vi "UMLEditor_PackageClasses.vi"(0 "DiagramIn":refnum<class "Graph.lvclass">, 3 "Settings":T1={"Levels"=-1}, 5 "error in (no error)":errorcluster) -> (19 "error out":errorcluster)   [LabVIEW 2020]
doc: "Gets current diagram values"
uses:
  <resource>/Framework/Providers/Open_GDS/UML/UMLEditor/UMLEditor_PackageClasses.ctl
  <resource>/Framework/Providers/Open_GDS/UML/Graph_class/Graph.lvclass
  <resource>/Framework/Providers/Open_GDS/UML/Graphics_class/FontType.ctl
  <resource>/Framework/Providers/Open_GDS/UML/UMLEditor/UMLEditor BusyDialogAction.ctl
  <resource>/Framework/Providers/Open_GDS/UML/ClassNode_class/ClassNode.lvclass
  C:/Program Files (x86)/National Instruments/LabVIEW 2020/resource/Framework/Providers/Open_GDS/UML/AbstractNode_class/AbstractNode.lvclass
  <resource>/Framework/Providers/Open_GDS/UML/PackageNode_class/PackageNode.lvclass
  C:/Program Files (x86)/National Instruments/LabVIEW 2020/resource/Framework/Providers/Open_GDS/UML/RectangularNode_class/RectangularNode.lvclass
  <resource>/Framework/Providers/Open_GDS/UML/ContextHelp/ContextHelp_HelpTexts.ctl
  <resource>/Framework/Providers/Open_GDS/UML/General/Point/Point Point2D.ctl
  <resource>/Framework/Providers/Open_GDS/UML/RectangularNode_class/RectangularNode.lvclass
  <resource>/Framework/Providers/Open_GDS/UML/Graphics_class/Graphics.lvclass
  <resource>/Framework/Providers/Open_GDS/UML/AbstractNode_class/AbstractNode.lvclass
panel:
  in  "MoveNodes":bool
  in  "Levels":i32=3 caption="Maximum levels of packages to create" min=1 max=100
  in  "Help":bool
  in  "cancel":bool
  in  "ok":bool
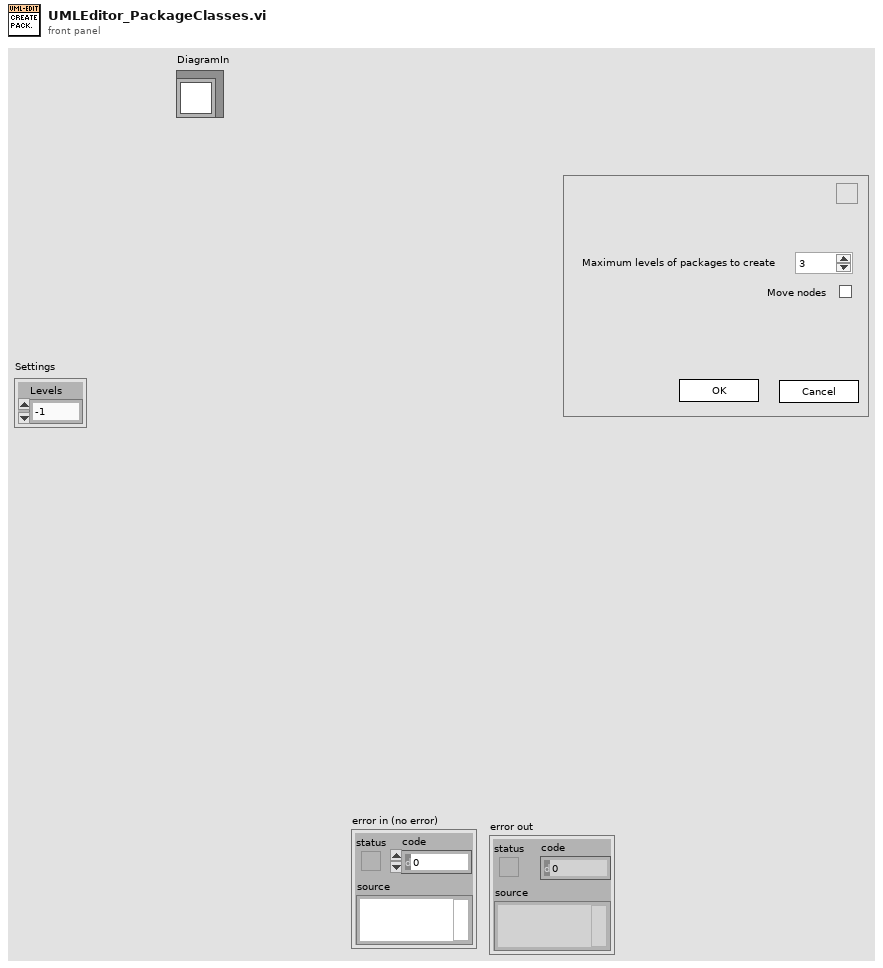
[diagram p1: front panel]
types:
  T1 = typedef "UMLEditor_PackageClasses.ctl" = cluster{"Levels":i32}
  T2 = cluster{"ClassNodes":refnum<class "ClassNode.lvclass">[], "Folders":cluster{"Foldername":string, "Path":path, "Nodes":refnum<class "ClassNode.lvclass">[], "SubFolders":path[], "PackageNode":refnum<class "PackageNode.lvclass">}[], "PackageNames":string[], "PackagesNodes":refnum<class "PackageNode.lvclass">[]}
  T3 = typedef "UMLEditor BusyDialogAction.ctl" = enum16{"Initialize", "Open(VIs)", "Open(i)", "Send_I-Value", "SendStatusMessage", "GetBusyDialogStatus", "Close", "Quit"}
  T4 = typedef "Graphics.lvclass/FontType.ctl" = cluster{"Font Name:":string, "Size":i16, "Strikeout?":bool, "Italic?":bool, "Underline?":bool, "Outline?":bool, "Shadow?":bool, "Bold?":bool}
  T5 = typedef "ContextHelp_HelpTexts.ctl" = enum16{"None(Hide)", "Default", "Help", "Welcome", "GettingStarted", "ClassDiagram_Help", "SequenceDiagram_Help", "UseCaseDiagram_Help", "BSelect", "BClass", "BInterface", "BPackage", "BNote", "BDependency", "BInheritance", "BInterfaceImplementation", "BAssociation", "BAggregation", "BCompAggregation", "BNoteConnector", "BObject", "BActionBar", "BCall", "BSystem", "BActor", "BUseCase", "BGeneralization", "BIncludes", "BExtends", "BUseCaseDiagramAssociation", "ClassRelationshipEdge editDialog_Bent Style", "ClassRelationshipEdge editDialog_RelationType", "ClassRelationshipEdge editDialog_Reverse association", "ClassRelationshipEdge editDialog_Start label", "ClassRelationshipEdge editDialog_Middle label", "ClassRelationshipEdge editDialog_End label", "UMLEditor reversedEngineering_Pathes", "ReversedEngineering StateReverseDialog_Help", "ReversedEngineering StateQueuedSettings_Help", "UMLEditor reversedEngineering_AddTopVIs", "UMLEditor reversedEngineering_AddClasses", "UMLEditor reversedEngineering_AddDirs", "UMLEditor reversedEngineering_Recursively", "UMLEditor reversedEngineering_Remove", "UMLEditor reversedEngineering_ClearList", "UMLEditor reversedEngineering_HideSubAss", "UMLEditor reversedEngineering_CreateTypes", "UMLEditor reversedEngineering_OnlyInheritance", "UMLEditor reversedEngineering_CreateApplication", "UMLEditor reversedEngineering_OK", "UMLEditor reversedEngineering_Cancel", "UMLEditor reversedEngineering_Help", "UMLEditor createWizardScriptFile_ScriptfilePath", "UMLEditor createWizardScriptFile_ClassPath", "UMLEditor createWizardScriptFile_Use", "UMLEditor createWizardScriptFile_PrivateDirName", "UMLEditor createWizardScriptFile_DirAppend", "UMLEditor createWizardScriptFile_Separator Character", "UMLEditor createWizardScriptFile_OK", "UMLEditor createWizardScriptFile_Cancel", "UMLEditor createWizardScriptFile_Help", "ClassNode editDialog_Class Name", "InterfaceNode editDialog_Class Name", "ClassNode editDialog_Attribute", "ClassNode editDialog_Methods", "InterfaceNode editDialog_Methods", "ClassNode editDialog_connection", "InterfaceNode editDialog_connection", "ClassNode editDialog_StereoType", "ClassNode editDialog_ShowAttrib", "ClassNode editDialog_ShowMethods", "ClassNode editDialog_ClassPath", "ClassNode editDialog_AddAttribute", "ClassNode editDialog_AddMethod", "InterfaceNode editDialog_AddMethod", "ClassNode AttributeGuide_AttributeName", "ClassNode AttributeGuide_Array?", "ClassNode AttributeGuide_Data Type", "ClassNode AttributeGuide_RefName", "ClassNode AttributeGuide_Preview", "ClassNode AttributeGuide_OK", "ClassNode AttributeGuide_Cancel", "ClassNode MethodGuide_Visibility", "ClassNode MethodGuide_Method Name", "ClassNode MethodGuide_Preview", "ClassNode MethodGuide_OK", "ClassNode MethodGuide_Cancel", "CallNode EditCallProperties_AllButtons", "ObjectNode EditObjectlProperties_AllButtons", "ActorNode EditActorProperties_AllButtons", "UseCaseRelationshipNode EditUseCaselProperties_AllButtons", "UseCaseNode EditUseCaselProperties_AllButtons", "SystemNode EditSystemProperties_AllButtons", "ReversedEngineering UpdateAttributes_AllButtons", "StateNode editDialog_AllButtons", "StateTransition editDialog_AllButtons", "ArrangeNodes Main_Picture", "ArrangeNodes Main_Zoom", "ArrangeNodes Main_Auto Zoom", "ArrangeNodes Main_shorten", "ArrangeNodes Main_Min Length", "ArrangeNodes Main_Max Length", "ArrangeNodes Main_increase", "ArrangeNodes Main_decrease", "ArrangeNodes Main_Shake", "ArrangeNodes Main", "BState", "BInitialState", "BFinalState", "BStateTransition", "StateDiagram_Help", "StateDiagram_PropertiesAllButtons", "ReversedEngineering StateReverseDialog_ClearStates", "ReversedEngineering StateReverseDialog_UseQueuedStateMachines", "ReversedEngineering StateReverseDialog_QueuedSettings", "ReversedEngineering StateReverseDialog_SearchForVIs", "ReversedEngineering StateReverseDialog_SearchCriteria", "OptionsDialog_ClassBasePath", "OptionsDialog_VIPath", "OptionsDialog_ApplicationPath", "OptionsDialog_WizDir", "OptionsDialog_IniFilePath", "OptionsDialog_DefineColors", "OptionsDialog_Help", "OptionsDialog_CreateTypes", "ClassRelationshipEdge editDialog_SplitWire"}
  T6 = typedef "Point Point2D.ctl" = cluster{"x":dbl, "y":dbl}
  T7 = typedef "ContextHelp_ShowType.ctl" = cluster{"Header":string, "Picture":picture, "Text":string}
  T8 = cluster{"Foldername":string, "Path":path, "Nodes":refnum<class "ClassNode.lvclass">[], "SubFolders":path[], "PackageNode":refnum<class "PackageNode.lvclass">}
  T9 = cluster{"Foldername":string, "Path":path, "Nodes":refnum<class "ClassNode.lvclass">[], "SubFolders":path[], "PackageNode":refnum<class "PackageNode.lvclass">}[]
  T10 = typedef "Rectangle Rectangle2D.ctl" = cluster{"x":dbl, "y":dbl, "width":dbl, "height":dbl}
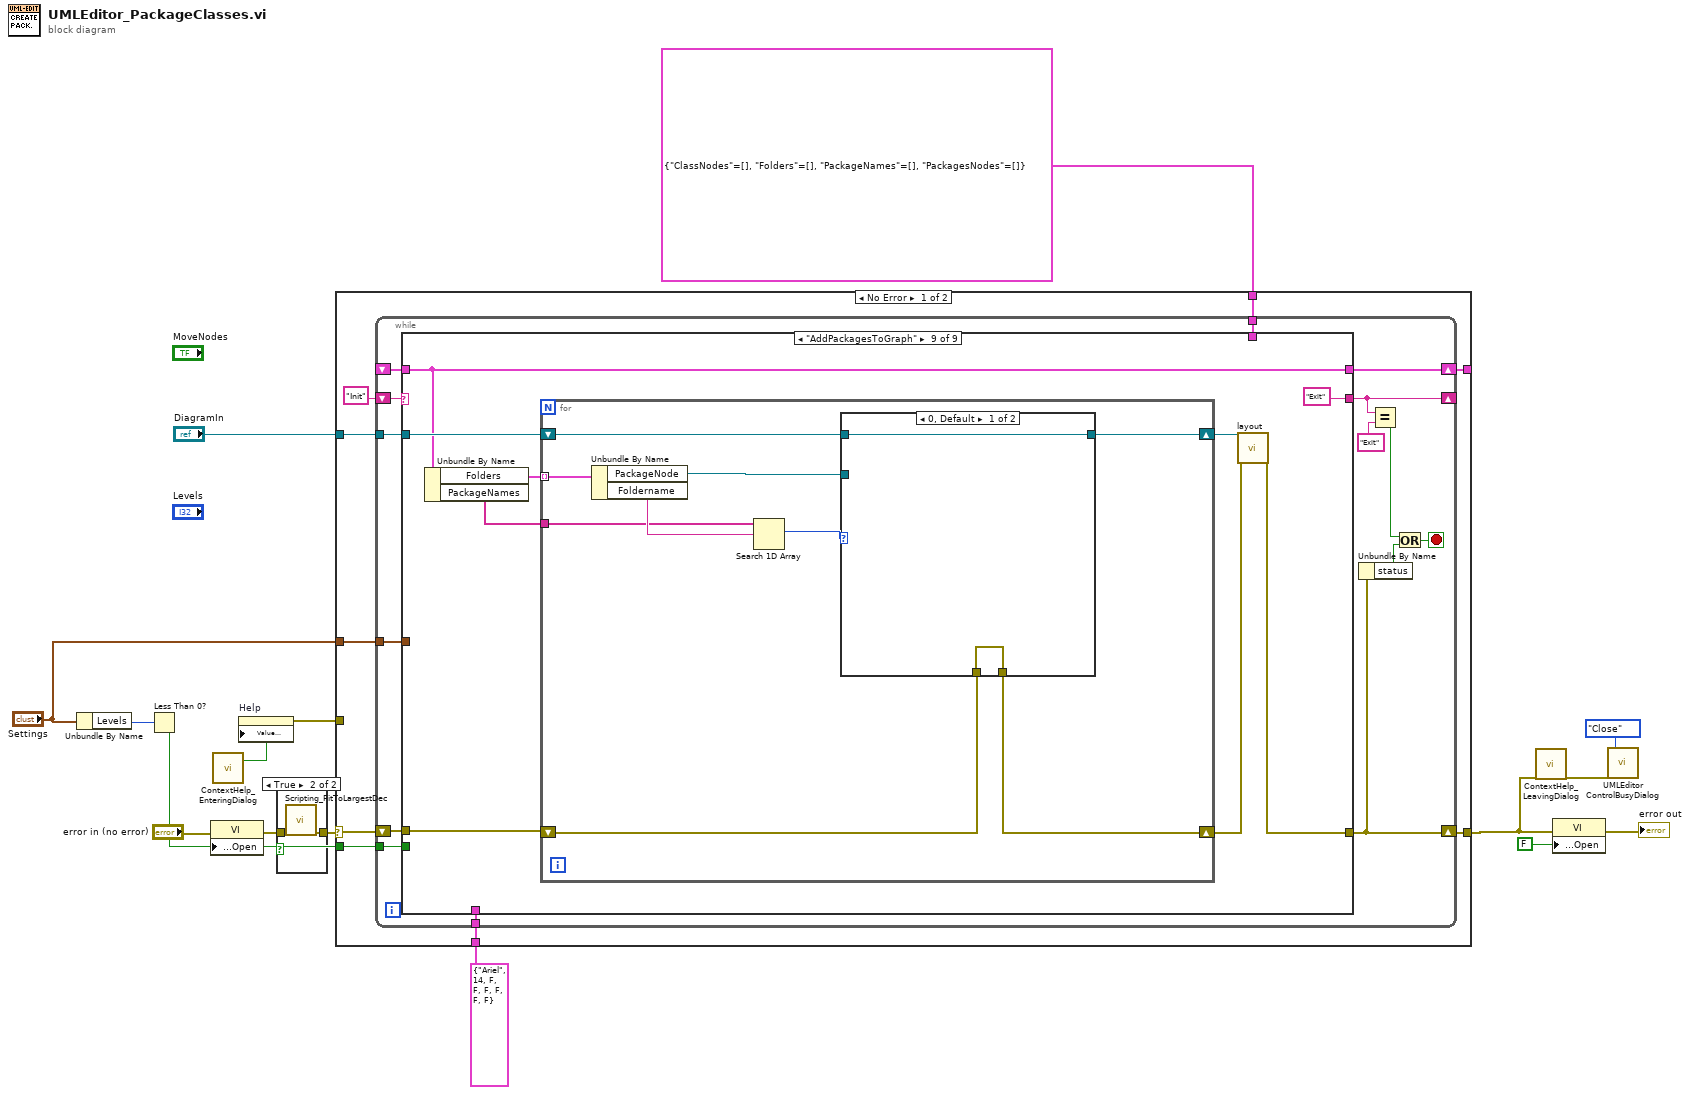
[diagram p0: block diagram]
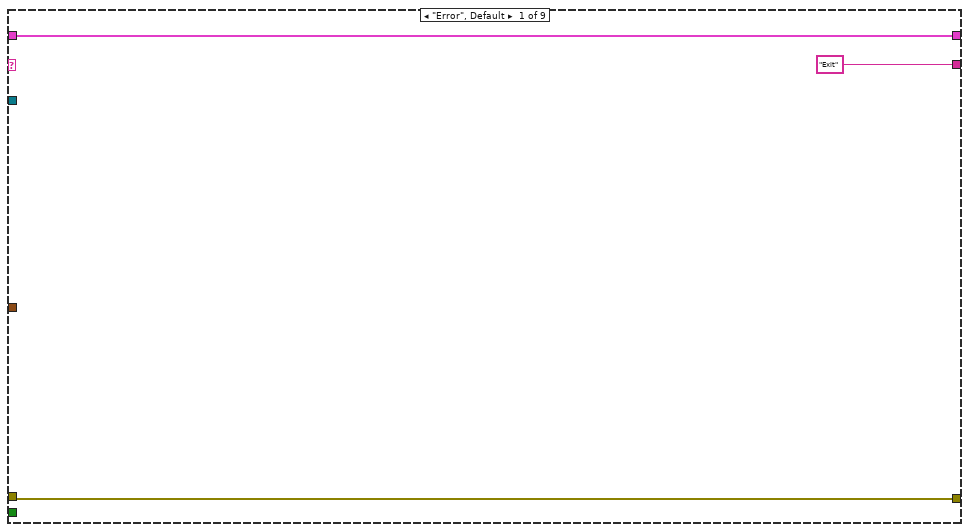
[diagram p3: hidden frame]
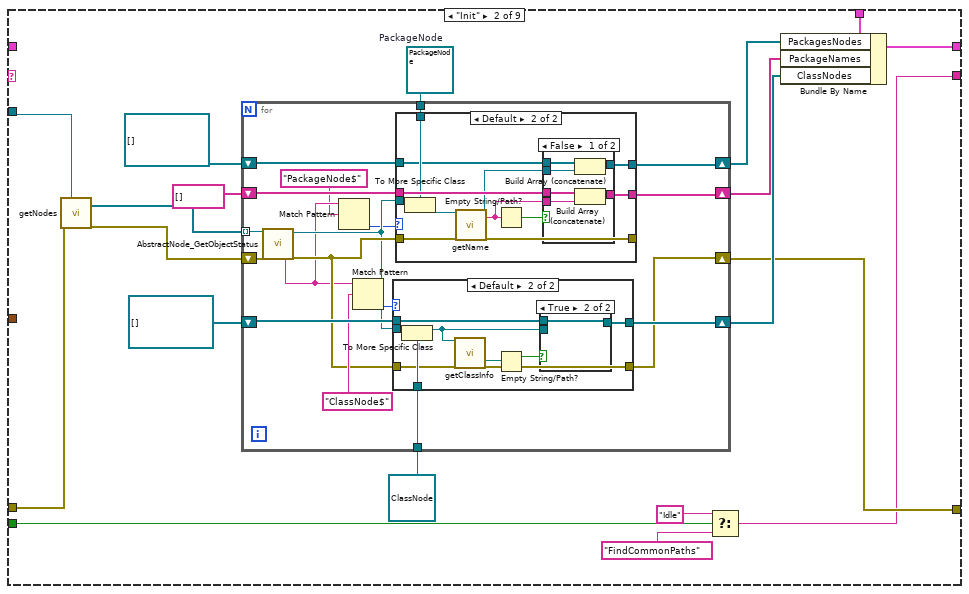
[diagram p4: hidden frame]
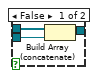
[diagram p8: hidden frame]
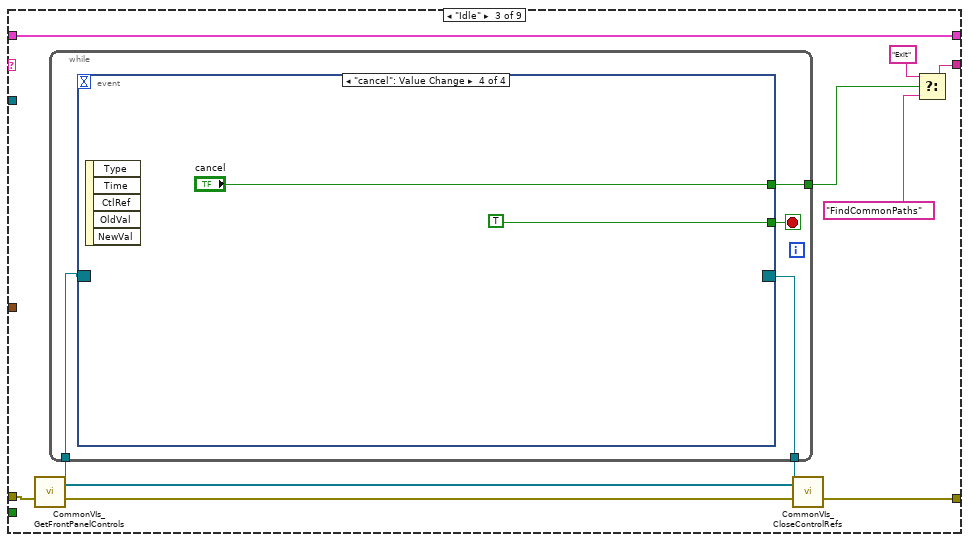
[diagram p9: hidden frame]
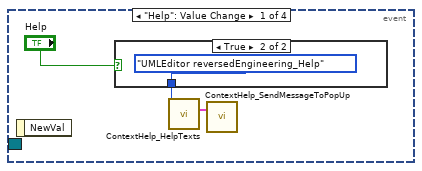
[diagram p10: hidden frame]
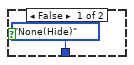
[diagram p11: hidden frame]
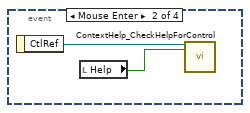
[diagram p12: hidden frame]
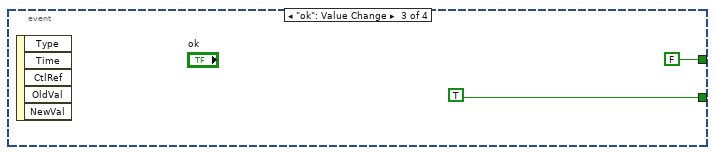
[diagram p13: hidden frame]
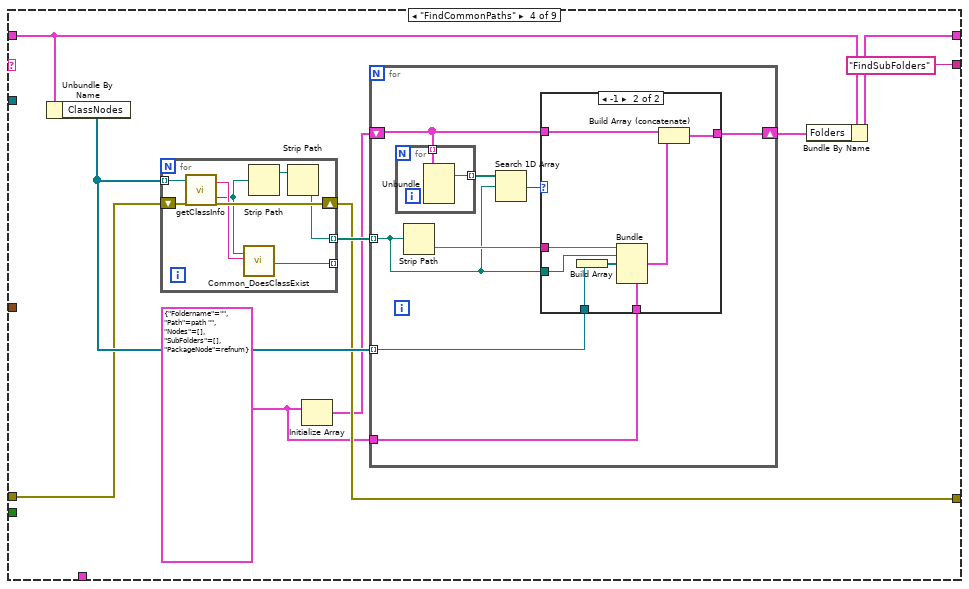
[diagram p14: hidden frame]
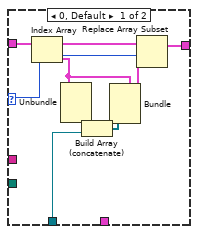
[diagram p15: hidden frame]
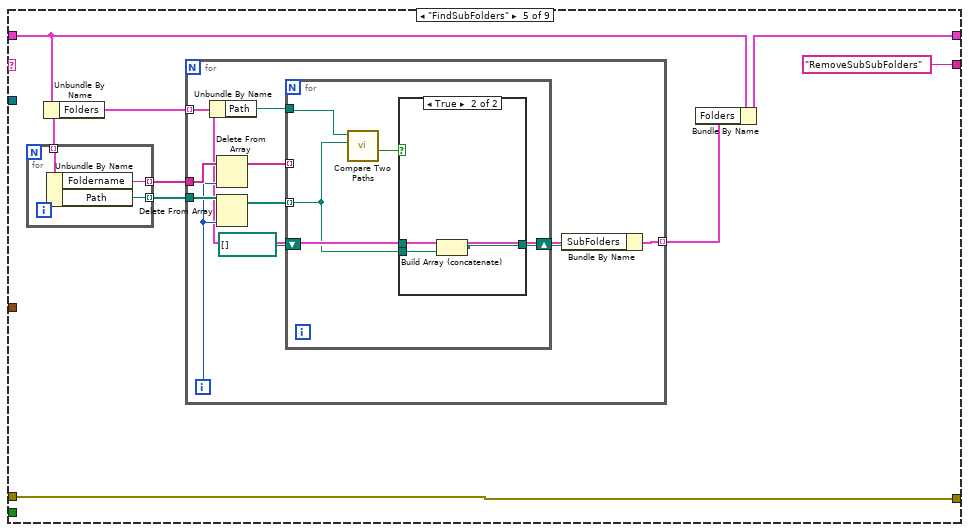
[diagram p16: hidden frame]
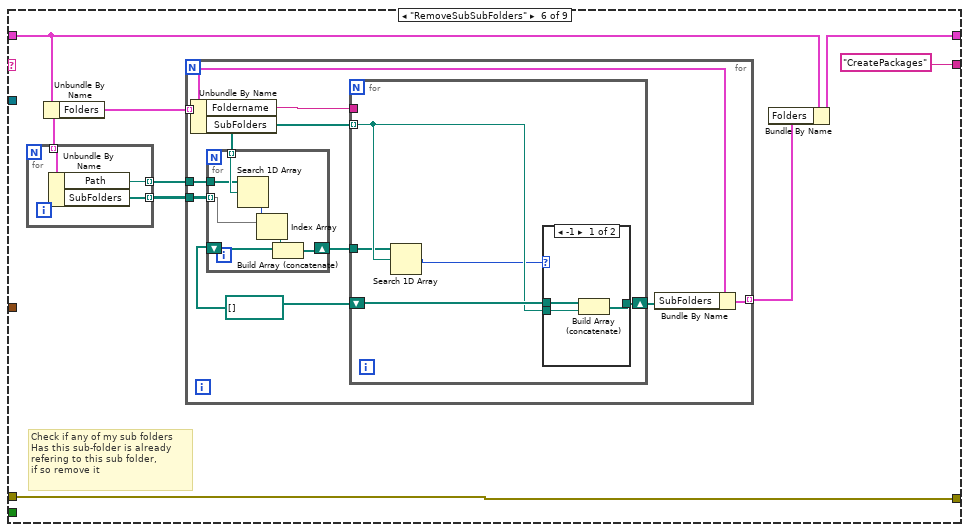
[diagram p18: hidden frame]
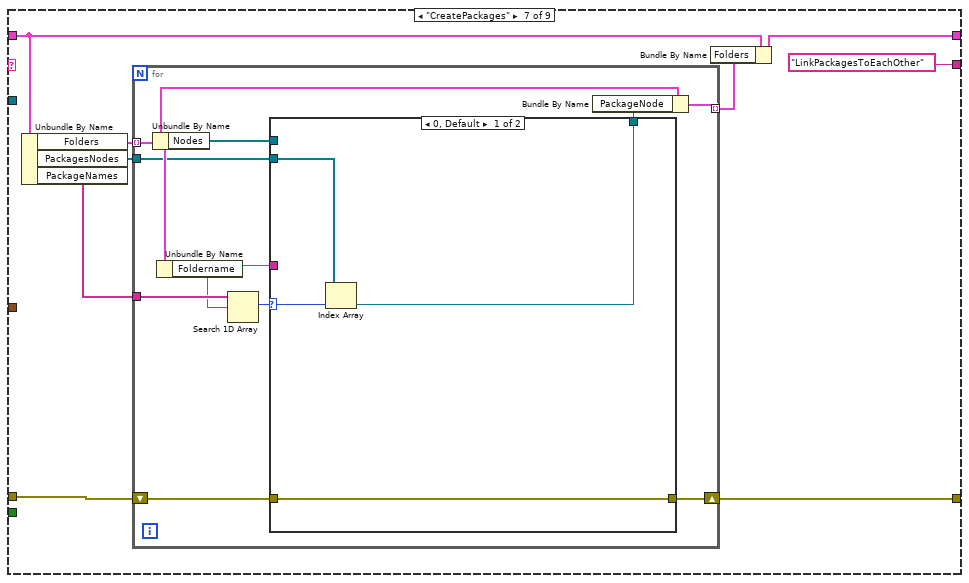
[diagram p20: hidden frame]
diagram:
  n1 = Unbundle By Name("Settings") -> ("Levels"=w5:i32)
  n2 = Less Than 0?(x=w5) -> (x < 0?=w4:bool)
  n3 = property class="VI"(error in="error in (no error)", "Front Panel.Open"=w4) -> (error out=w7:errorcluster)  [unwired: 1 in, 1 out]
  n4 = call <resource>:"ContextHelp_EnteringDialog.vi"() -> ("HelpStatus"=w16:bool)  [unwired: 1 in, 18 out]
  n5 = property on="Help" class="Bool (strict)"("Value (Signaling)"=w16) -> (error out=w15:errorcluster)  [unwired: 2 in, 1 out]
  n6 = case shown="True" w4 {
    tunnel: w7 -> [w17 w19]
    tunnel: [w17 w18] -> w6
    frame False {
    }
    frame True {
      n7 = call <resource>:"Scripting_FitToLargestDec.vi"("error in (no error)"=w19) -> ("error out"=w18:errorcluster)  [unwired: 5 in, 1 out]
    }
  }
  n8 = case shown="No Error" w6 {
    selector: w6 -> [w26 w374]
    tunnel: [w27 w374] -> w12
    tunnel: [w25 _] -> _
    tunnel: w15 -> [_ _]
    tunnel: T4 {"Font Name:"="Ariel", "Size"=14, "Strikeout?"=FALSE, "Italic?"=FALSE, "Underline?"=FALSE, "Outline?"=FALSE, "Shadow?"=FALSE, "Bold?"=FALSE} ("font") -> [w24 _]
    tunnel: w4 -> [w23 _]
    tunnel: T2 {"ClassNodes"=[], "Folders"=[], "PackageNames"=[], "PackagesNodes"=[]} ("local") -> [w22 _]
    tunnel: "Settings" -> [w21 _]
    tunnel: "DiagramIn" -> [w20 _]
    frame No Error {
      n9 = while {
        shift-right: [w40] -> w27
        shift-left: w26 -> [w29]
        shift-right: [w38] -> _
        shift-left: "Init" -> [w43]
        shift-right: [w42] -> w25
        shift-left: _ -> [w41]
        tunnel: w24 -> [w34]
        tunnel: w23 -> [w33]
        tunnel: w22 -> [w32]
        tunnel: w21 -> [w31]
        tunnel: w20 -> [w30]
        stop <- w35 stop-if-true
        n10 = case shown="\"AddPackagesToGraph\"" w43 {
          tunnel: [w44 w57 w122 w153 w196 w227 w259 w304 w350] -> w40
          tunnel: [w45 w60 w124 w148 w190 w221 w260 w309 w354] -> w42
          tunnel: ["Exit" w53 w129 "FindSubFolders" ("y") "RemoveSubSubFolders" ("y") "CreatePackages" ("y") "LinkPackagesToEachOther" ("y") "AddPackagesToGraph" ("y") "Exit" ("y")] -> w38
          tunnel: w41 -> [w45 _ w124 w149 w191 w222 w261 w309 w354]
          tunnel: w34 -> [_ _ _ _ _ _ _ _ _]
          tunnel: w33 -> [_ w56 _ _ _ _ _ _ _]
          tunnel: w32 -> [_ w61 _ _ _ _ _ _ _]
          tunnel: w31 -> [_ _ _ _ _ _ _ _ _]
          tunnel: w30 -> [_ w62 _ _ _ _ _ _ w355]
          tunnel: w29 -> [w44 w51 w122 w147 w196 w227 w258 w310 w349]
          frame "Error", Default {
          }
          frame "Init" {
            w50 = refnum<class "PackageNode.lvclass"> refnum  # PackageNode
            n11 = call-dynamic "getNodes.vi"("reference"=w62, "error in (no error)"=w51) -> ("nodes"=w59:refnum<class "AbstractNode.lvclass">[], "error out"=w64:errorcluster)  [unwired: 15 in, 1 out]
            n12 = for {
              shift-right: [w76] -> w57
              shift-left: w64 -> [w83]
              tunnel: w59 -> [w82] mode=indexing
              shift-right: [w80] -> w58
              shift-left: refnum<class "ClassNode.lvclass">[] [] -> [w81]
              tunnel: refnum<class "ClassNode.lvclass"> refnum ("reference out") -> [w77]
              shift-right: [w68] -> w49
              shift-left: string[] [] -> [w73]
              tunnel: w50 -> [w75]
              shift-right: [w67] -> w47
              shift-left: refnum<class "PackageNode.lvclass">[] [] -> [w66]
              n13 = call <resource>:"AbstractNode_GetObjectStatus.vi"("reference in"=w82, "error in (no error)"=w83) -> ("Class name"=w71:string, "reference out"=w72:refnum<class "AbstractNode.lvclass">, "error out"=w74:errorcluster)  [unwired: 15 out]
              n14 = Match Pattern(string=w71, regular expression="PackageNode$") -> (offset past match=w69:i32)  [unwired: 4 out]
              n15 = Match Pattern(string=w71, regular expression="ClassNode$") -> (offset past match=w78:i32)  [unwired: 4 out]
              n16 = case shown="Default" w78 {
                tunnel: w81 -> [w108 w117]
                tunnel: w72 -> [_ w115]
                tunnel: [w108 w116] -> w80
                tunnel: w77 -> [_ w114]
                tunnel: w74 -> [w107 w112]
                tunnel: [w107 w109] -> w76
                frame -1 {
                }
                frame Default {
                  n17 = To More Specific Class(target class=w114, reference=w115) -> (specific class reference=w113:refnum<class "ClassNode.lvclass">)  [unwired: 1 in, 1 out]
                  n18 = call-dynamic "getClassInfo.vi"("reference"=w113, "error in (no error)"=w112) -> ("ClassPath"=w111:path, "error out"=w109:errorcluster)  [unwired: 8 in, 8 out]
                  n19 = Empty String/Path?(string/path=w111) -> (empty?=w110:bool)
                  n20 = case shown="True" w110 {
                    tunnel: w117 -> [w120 w121]
                    tunnel: [w119 w121] -> w116
                    tunnel: w113 -> [w118 _]
                    frame False {
                      n21 = Build Array (concatenate)(w120, w118) -> (w119:refnum<class "ClassNode.lvclass">[])
                    }
                    frame True {
                    }
                  }
                }
              }
              n22 = case shown="Default" w69 {
                tunnel: w73 -> [w86 w98]
                tunnel: w72 -> [_ w96]
                tunnel: [w86 w97] -> w68
                tunnel: w74 -> [w85 w92]
                tunnel: [w85 w90] -> _
                tunnel: w75 -> [_ w94]
                tunnel: [w84 w89] -> w67
                tunnel: w66 -> [w84 w88]
                frame -1 {
                }
                frame Default {
                  n23 = To More Specific Class(target class=w94, reference=w96) -> (specific class reference=w93:refnum<class "PackageNode.lvclass">)  [unwired: 1 in, 1 out]
                  n24 = call-dynamic "getName.vi"("reference"=w93, "error in (no error)"=w92) -> ("reference out"=w87:refnum<class "PackageNode.lvclass">, "name"=w91:string, "error out"=w90:errorcluster)  [unwired: 15 in]
                  n25 = Empty String/Path?(string/path=w91) -> (empty?=w95:bool)
                  n26 = case shown="False" w95 {
                    tunnel: w98 -> [w101 w106]
                    tunnel: [w104 w106] -> w97
                    tunnel: w91 -> [w103 _]
                    tunnel: [w102 w105] -> w89
                    tunnel: w88 -> [w100 w105]
                    tunnel: w87 -> [w99 _]
                    frame False {
                      n27 = Build Array (concatenate)(w100, w99) -> (w102:refnum<class "PackageNode.lvclass">[])
                      n28 = Build Array (concatenate)(w101, w103) -> (w104:string[])
                    }
                    frame True {
                    }
                  }
                }
              }
            }
            n29 = Select(t="Idle" ("y"), s=w56, f="FindCommonPaths") -> (s? t:f=w53:string)
            n30 = Bundle By Name(cluster=w61, "PackagesNodes"=w47, "PackageNames"=w49, "ClassNodes"=w58) -> (w60:T2)
          }
          frame "Idle" {
            n31 = call <resource>:"CommonVIs_GetFrontPanelControls.vi"() -> ("Event Registration Refnum"=w127:refnum<event-registration>, "ControlRefs"=w125:refnum<vi>[])  [unwired: 2 in, 16 out]
            n32 = while {
              tunnel: [w134] -> w123
              tunnel: w127 -> [w132]
              tunnel: [w131] -> w126
              stop <- w133 stop-if-true
              n33 = event shown="[3] \"cancel\": Value Change" {
                selector: w132 -> [_ _ _ _]
                dyn-events: [_ _ _ _] -> w131
                timeout: _ -> [_ _ _ _]
                tunnel: [_ _ FALSE ("cancel") "cancel"] -> w134
                tunnel: [_ _ TRUE ("Front Panel Window:Is Frontmost") TRUE ("Front Panel Window:Is Frontmost")] -> w133
                event "Help": Value Change {
                  n34 = event-data() -> ()  [unwired: 2 out]
                  n35 = case shown="True" "Help" {
                    tunnel: [ContextHelp_HelpTexts."None(Hide)" ("HelpText") ContextHelp_HelpTexts."UMLEditor reversedEngineering_Help" ("HelpText")] -> w136
                    frame False {
                    }
                    frame True {
                    }
                  }
                  n36 = call <resource>:"ContextHelp_HelpTexts.vi"("HelpText (enum or string)"=w136) -> ("HelpOut"=w137:T7)  [unwired: 18 out]
                  n37 = call <resource>:"ContextHelp_SendMessageToPopUp.vi"("PopUpMessage"=w137) -> ()  [unwired: 2 in, 17 out]
                }
                event Mouse Enter {
                  n38 = event-data() -> ("CtlRef"=w141:refnum<vi>)  [unwired: 1 out]
                  n39 = local read "Help"() -> (w140:bool)
                  n40 = call <resource>:"ContextHelp_CheckHelpForControl.vi"("Ctl Refnum"=w141, "Help"=w140) -> ()  [unwired: 1 in, 17 out]
                }
                event "ok": Value Change {
                  n41 = event-data() -> ()  [unwired: 6 out]
                }
                event "cancel": Value Change {
                  n42 = event-data() -> ()  [unwired: 6 out]
                }
              }
            }
            n43 = call <resource>:"CommonVIs_CloseControlRefs.vi"("Event Registration Refnum"=w126, "ControlRefs"=w125) -> ()  [unwired: 1 in, 17 out]
            n44 = Select(t="Exit", s=w123, f="FindCommonPaths") -> (s? t:f=w129:string)
          }
          frame "FindCommonPaths" {
            w151 = T8 {"Foldername"="", "Path"=path "", "Nodes"=[], "SubFolders"=[], "PackageNode"=refnum}
            n45 = Unbundle By Name(w149) -> ("ClassNodes"=w155:refnum<class "ClassNode.lvclass">[])
            n46 = for {
              tunnel: w155 -> [w189] mode=indexing
              shift-right: [w187] -> w153
              shift-left: w147 -> [w188]
              tunnel: [w182] -> w154 mode=indexing
              tunnel: [w185] -> _ mode=indexing
              n47 = call-dynamic "getClassInfo.vi"("reference"=w189, "error in (no error)"=w188) -> ("className"=w186:string, "ClassPath"=w183:path, "error out"=w187:errorcluster)  [unwired: 8 in, 7 out]
              n48 = call <resource>:"Common_DoesClassExist.vi"("ClassPath"=w183, "ClassName"=w186) -> ("llb/LvCLass-Path"=w185:path)  [unwired: 17 out]
              n49 = Strip Path(path=w183) -> (stripped path=w184:path)  [unwired: 1 out]
              n50 = Strip Path(path=w184) -> (stripped path=w182:path)  [unwired: 1 out]
            }
            n51 = Initialize Array(w151) -> (w152:T9)  [unwired: 1 in]
            n52 = for {
              tunnel: w154 -> [w156] mode=indexing
              tunnel: w155 -> [w158] mode=indexing
              shift-right: [w163] -> w146
              shift-left: w152 -> [w161]
              tunnel: w151 -> [w157]
              n53 = for {
                tunnel: [w180] -> w162 mode=indexing
                tunnel: w161 -> [w181] mode=indexing
                n54 = Unbundle(w181) -> ("Path"=w180:path)  [unwired: 4 out]
              }
              n55 = Strip Path(path=w156) -> (name=w160:string)  [unwired: 1 out]
              n56 = Search 1D Array(1D array=w162, element=w156) -> (index of element=w159:i32)  [unwired: 1 in]
              n57 = case shown="-1" w159 {
                selector: w159 -> [w168 _]
                tunnel: w156 -> [_ w179]
                tunnel: [w167 w178] -> w163
                tunnel: w161 -> [w169 w177]
                tunnel: w160 -> [_ w176]
                tunnel: w158 -> [w170 w175]
                tunnel: w157 -> [_ w174]
                frame 0, Default {
                  n58 = Index Array(array=w169, index=w168) -> (element=w166:T8)
                  n59 = Unbundle(w166) -> ("Nodes"=w171:refnum<class "ClassNode.lvclass">[])  [unwired: 4 out]
                  n60 = Build Array (concatenate)(w171, w170) -> (w165:refnum<class "ClassNode.lvclass">[])
                  n61 = Bundle(cluster=w166, "Nodes"=w165) -> (w164:T8)  [unwired: 4 in]
                  n62 = Replace Array Subset(array=w169, new element=w164, index=w168) -> (w167:T9)
                }
                frame -1 {
                  n63 = Build Array(w175) -> (w173:refnum<class "ClassNode.lvclass">[])
                  n64 = Bundle(cluster=w174, "Foldername"=w176, "Path"=w179, "Nodes"=w173) -> (w172:T8)  [unwired: 2 in]
                  n65 = Build Array (concatenate)(w177, w172) -> (w178:T9)
                }
              }
            }
            n66 = Bundle By Name(cluster=w149, "Folders"=w146) -> (w148:T2)
          }
          frame "FindSubFolders" {
            n67 = Unbundle By Name(w191) -> ("Folders"=w195:T9)
            n68 = for {
              tunnel: w195 -> [w200] mode=indexing
              tunnel: [w199] -> w193 mode=indexing
              tunnel: [w198] -> w194 mode=indexing
              n69 = Unbundle By Name(w200) -> ("Foldername"=w199:string, "Path"=w198:path)
            }
            n70 = for {
              tunnel: w195 -> [w204] mode=indexing
              tunnel: w194 -> [w210]
              tunnel: w193 -> [w209]
              tunnel: [w202] -> w192 mode=indexing
              i -> [w208]
              n71 = Unbundle By Name(w204) -> ("Path"=w207:path)
              n72 = Delete From Array(array=w209, index=w208) -> (array with subset deleted=w205:string[])  [unwired: 1 in, 1 out]
              n73 = Delete From Array(array=w210, index=w208) -> (array with subset deleted=w206:path[])  [unwired: 1 in, 1 out]
              n74 = for {
                tunnel: w207 -> [w215]
                tunnel: w206 -> [w211] mode=indexing
                shift-right: [w212] -> w203
                shift-left: path[] [] -> [w213]
                tunnel: w205 -> [_] mode=indexing
                n75 = call <vilib>:"Compare Two Paths.vi"("Path 2"=w211, "Path 1"=w215) -> ("Path 2 Relative to Path 1?"=w214:bool)  [unwired: 6 in, 3 out]
                n76 = case shown="True" w214 {
                  tunnel: w213 -> [w216 w219]
                  tunnel: w211 -> [_ w218]
                  tunnel: [w216 w217] -> w212
                  frame False {
                  }
                  frame True {
                    n77 = Build Array (concatenate)(w219, w218) -> (w217:path[])
                  }
                }
              }
              n78 = Bundle By Name(cluster=w204, "SubFolders"=w203) -> (w202:T8)
            }
            n79 = Bundle By Name(cluster=w191, "Folders"=w192) -> (w190:T2)
          }
          frame "RemoveSubSubFolders" {
            # "Check if any of my sub folders\nHas this sub-folder is already \nrefering to this sub folder,\nif so remove it"
            n80 = Unbundle By Name(w222) -> ("Folders"=w226:T9)
            n81 = for {
              tunnel: w226 -> [w230] mode=indexing
              tunnel: [w229] -> w224 mode=indexing
              tunnel: [w228] -> w225 mode=indexing
              n82 = Unbundle By Name(w230) -> ("Path"=w229:path, "SubFolders"=w228:path[])
            }
            n83 = for {
              tunnel: w226 -> [w238] mode=indexing
              tunnel: w225 -> [w233]
              tunnel: w224 -> [w235]
              tunnel: [w236] -> w223 mode=indexing
              w232 = path[] []
              n84 = Unbundle By Name(w238) -> ("Foldername"=w239:string, "SubFolders"=w234:path[])
              n85 = for {
                tunnel: w234 -> [w246] mode=indexing
                tunnel: w235 -> [w240]
                tunnel: w233 -> [w245] mode=indexing
                shift-right: [w241] -> w231
                shift-left: w232 -> [w243]
                n86 = Search 1D Array(1D array=w240, element=w246) -> (index of element=w244:i32)  [unwired: 1 in]
                n87 = Index Array(array=w245, index=w244) -> (element=w242:path)
                n88 = Build Array (concatenate)(w243, w242) -> (w241:path[])
              }
              n89 = for {
                tunnel: w239 -> [_]
                shift-right: [w250] -> w237
                shift-left: w232 -> [w251]
                tunnel: w234 -> [w249] mode=indexing
                tunnel: w231 -> [w248]
                n90 = Search 1D Array(1D array=w248, element=w249) -> (index of element=w247:i32)  [unwired: 1 in]
                n91 = case shown="-1" w247 {
                  tunnel: w251 -> [w254 w255]
                  tunnel: [w253 w255] -> w250
                  tunnel: w249 -> [w252 _]
                  frame -1 {
                    n92 = Build Array (concatenate)(w254, w252) -> (w253:path[])
                  }
                  frame Default {
                  }
                }
              }
              n93 = Bundle By Name(cluster=w238, "SubFolders"=w237) -> (w236:T8)
            }
            n94 = Bundle By Name(cluster=w222, "Folders"=w223) -> (w221:T2)
          }
          frame "CreatePackages" {
            n95 = Unbundle By Name(w261) -> ("Folders"=w263:T9, "PackagesNodes"=w256:refnum<class "PackageNode.lvclass">[], "PackageNames"=w257:string[])
            n96 = for {
              tunnel: w263 -> [w272] mode=indexing
              shift-right: [w270] -> w259
              shift-left: w258 -> [w274]
              tunnel: [w269] -> w262 mode=indexing
              tunnel: w257 -> [w268]
              tunnel: w256 -> [w265]
              n97 = Unbundle By Name(w272) -> ("Nodes"=w273:refnum<class "ClassNode.lvclass">[])
              n98 = Unbundle By Name(w272) -> ("Foldername"=w267:string)
              n99 = Search 1D Array(1D array=w268, element=w267) -> (index of element=w266:i32)  [unwired: 1 in]
              n100 = case shown="0, Default" w266 {
                selector: w266 -> [w277 _]
                tunnel: w274 -> [w278 w293]
                tunnel: w273 -> [_ w287]
                tunnel: [w275 w281] -> w271
                tunnel: [w278 w280] -> w270
                tunnel: w267 -> [_ w279]
                tunnel: w265 -> [w276 _]
                frame 0, Default {
                  n101 = Index Array(array=w276, index=w277) -> (element=w275:refnum<class "PackageNode.lvclass">)
                }
                frame -1 {
                  n102 = Index Array(array=w287) -> (element=w294:refnum<class "ClassNode.lvclass">)  [unwired: 1 in]
                  n103 = call-dynamic "getBounds.vi"("reference"=w294, "error in (no error)"=w293) -> ("bounds"=w291:T10, "error out"=w292:errorcluster)  [unwired: 15 in, 1 out]
                  n104 = call <resource>:"PackageNode_Create.vi"("error in (no error)"=w292) -> ("reference out"=w296:refnum<class "PackageNode.lvclass">, "error out"=w295:errorcluster)  [unwired: 17 in]
                  n105 = Unbundle By Name(w291) -> ("x"=w289:dbl, "y"=w288:dbl)
                  n106 = call-dynamic "setName.vi"("reference"=w296, "name"=w279, "error in (no error)"=w295) -> ("reference out"=w285:refnum<class "PackageNode.lvclass">, "error out"=w286:errorcluster)  [unwired: 15 in]
                  n107 = Bundle By Name(cluster=T6 {"x"=0.0, "y"=0.0} ("point"), "x"=w289, "y"=w288) -> (w282:T6)
                  n108 = call <resource>:"setPosition.vi"("reference"=w285, "pos"=w282, "error in (no error)"=w286) -> ("reference out"=w284:refnum<class "PackageNode.lvclass">, "error out"=w283:errorcluster)  [unwired: 2 in, 13 out]
                  n109 = for {
                    shift-right: [w300] -> w280
                    shift-left: w283 -> [w301]
                    shift-right: [w298] -> w281
                    shift-left: w284 -> [w299]
                    tunnel: w287 -> [w297] mode=indexing
                    n110 = call-dynamic "addChild.vi"("reference"=w299, "node"=w297, "error in (no error)"=w301) -> ("reference out"=w298:refnum<class "PackageNode.lvclass">, "error out"=w300:errorcluster)  [unwired: 15 in]
                  }
                }
              }
              n111 = Bundle By Name(cluster=w272, "PackageNode"=w271) -> (w269:T8)
            }
            n112 = Bundle By Name(cluster=w261, "Folders"=w262) -> (w260:T2)
          }
          frame "LinkPackagesToEachOther" {
            n113 = Unbundle By Name(w309) -> ("Folders"=w308:T9)
            n114 = for {
              tunnel: w308 -> [w321] mode=indexing
              tunnel: [w320] -> w307 mode=indexing
              tunnel: [w319] -> w306 mode=indexing
              n115 = Unbundle By Name(w321) -> ("Path"=w320:path, "PackageNode"=w319:refnum<class "PackageNode.lvclass">)
            }
            n116 = for {
              tunnel: w308 -> [w331] mode=indexing
              shift-right: [w330] -> w305
              shift-left: w310 -> [w324]
              tunnel: w307 -> [w329]
              tunnel: w306 -> [w327]
              tunnel: [w322] -> w303 mode=indexing
              i -> [w328]
              n117 = Unbundle By Name(w331) -> ("PackageNode"=w322:refnum<class "PackageNode.lvclass">)
              n118 = Unbundle By Name(w331) -> ("SubFolders"=w326:path[])
              n119 = Delete From Array(array=w329, index=w328) -> (array with subset deleted=w325:path[])  [unwired: 1 in, 1 out]
              n120 = Delete From Array(array=w327, index=w328) -> (array with subset deleted=w323:refnum<class "PackageNode.lvclass">[])  [unwired: 1 in, 1 out]
              n121 = for {
                shift-right: [w337] -> w330
                shift-left: w324 -> [w338]
                tunnel: w326 -> [w335] mode=indexing
                tunnel: w325 -> [w336]
                tunnel: w323 -> [w333]
                tunnel: w322 -> [w332]
                n122 = Search 1D Array(1D array=w336, element=w335) -> (index of element=w334:i32)  [unwired: 1 in]
                n123 = case shown="Default" w334 {
                  selector: w334 -> [w340 _]
                  tunnel: w338 -> [w345 w346]
                  tunnel: [w344 w346] -> w337
                  tunnel: w332 -> [w343 w347]
                  tunnel: [w342 w347] -> _
                  tunnel: w333 -> [w341 _]
                  frame Default {
                    n124 = Index Array(array=w341, index=w340) -> (element=w339:refnum<class "PackageNode.lvclass">)
                    n125 = call-dynamic "addChild.vi"("reference"=w343, "node"=w339, "error in (no error)"=w345) -> ("reference out"=w342:refnum<class "PackageNode.lvclass">, "error out"=w344:errorcluster)  [unwired: 15 in]
                  }
                  frame -1 {
                  }
                }
              }
            }
            n126 = for {
              N: 10 -> [_]
              tunnel: w303 -> [w312]
              shift-right: [w313] -> w304
              shift-left: w305 -> [w314]
              n127 = for {
                tunnel: w312 -> [w315] mode=indexing
                shift-right: [w316] -> w313
                shift-left: w314 -> [w317]
                n128 = call-dynamic "ExecuteMenuCommand.vi"("reference"=w315, "Command"="Size to fit", "error in (no error)"=w317) -> ("error out"=w316:errorcluster)  [unwired: 13 in, 3 out]
              }
            }
          }
          frame "AddPackagesToGraph" {
            n129 = Unbundle By Name(w354) -> ("Folders"=w353:T9, "PackageNames"=w348:string[])
            n130 = for {
              tunnel: w353 -> [w362] mode=indexing
              shift-right: [w363] -> w351
              shift-left: w349 -> [w361]
              shift-right: [w364] -> w352
              shift-left: w355 -> [w365]
              tunnel: w348 -> [w358]
              n131 = Unbundle By Name(w362) -> ("PackageNode"=w360:refnum<class "PackageNode.lvclass">, "Foldername"=w359:string)
              n132 = Search 1D Array(1D array=w358, element=w359) -> (index of element=w357:i32)  [unwired: 1 in]
              n133 = case shown="0, Default" w357 {
                tunnel: w365 -> [w367 w373]
                tunnel: [w367 w372] -> w364
                tunnel: [w366 w371] -> w363
                tunnel: w361 -> [w366 w369]
                tunnel: w360 -> [_ w368]
                frame 0, Default {
                }
                frame -1 {
                  n134 = call-dynamic "addNode.vi"("reference"=w373, "node"=w368, "point"=T6 {"x"=nan, "y"=nan}, "error in (no error)"=w369) -> ("reference out"=w372:refnum<class "Graph.lvclass">, "error out"=w371:errorcluster)  [unwired: 14 in]
                }
              }
            }
            n135 = call-dynamic "layout.vi"("reference"=w352, "error in (no error)"=w351) -> ("error out"=w350:errorcluster)  [unwired: 16 in, 1 out]
          }
        }
        n136 = Unbundle By Name(w40) -> ("status"=w39:bool)
        n137 = Equal?(x=w38, y="Exit") -> (x = y?=w36:bool)
        n138 = Or(x=w36, y=w39) -> (x .or. y?=w35:bool)
      }
    }
    frame Error {
    }
  }
  n139 = call <resource>:"ContextHelp_LeavingDialog.vi"("error in (no error)"=w12) -> ("error out"=w8:errorcluster)  [unwired: 18 out]
  n140 = property class="VI"(error in=w12, "Front Panel.Open"=FALSE ("Front Panel Window:Open")) -> (error out=→"error out":errorcluster)  [unwired: 1 in, 1 out]
  n141 = call <resource>:"UMLEditor ControlBusyDialog.vi"("error in (no error)"=w8, "Action(SendStatusMessage)"=UMLEditor_BusyDialogAction."Close" ("Action")) -> ()  [unwired: 2 in, 16 out]
